vi "Validate Sequence File.vi"(10 "Path":path) -> (1 "Test Sequence":T1[](array[typedef]), 3 "Valid?":bool)   [LabVIEW 2015]
uses:
  Test Sequence Action.ctl
  Valve Action Enum.ctl
  Sequence File IO/Test Sequence Trigger.ctl
  Sequence File IO/Single Test Sequence.ctl
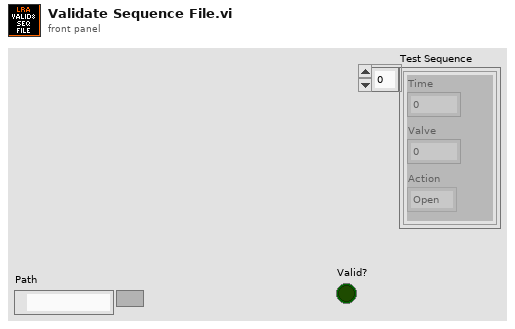
[diagram p1: front panel]
types:
  T1 = typedef "Test Sequence Action.ctl" = cluster{"Time":u32, "Valve":u32, "Action":T2}
  T2 = typedef "Valve Action Enum.ctl" = enum16{"Open", "Close"}
  T3 = typedef "Single Test Sequence.ctl" = cluster{"Actions":T1[], "Triggers":T4[]}
  T4 = typedef "Test Sequence Trigger.ctl" = cluster{"Begin Time (ms)":dbl, "End Time(ms)":dbl, "Sensor":enum16{""}, "Min Value":dbl, "Max Value":dbl}
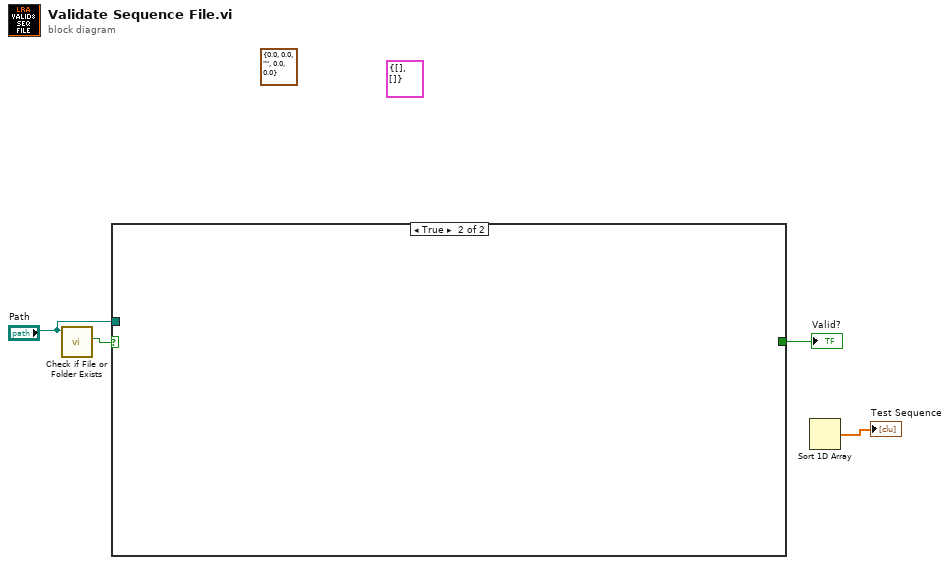
[diagram p0: block diagram]
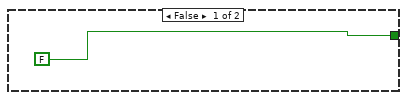
[diagram p2: hidden frame]
diagram:
  (unwired) T3 {"Actions"=[], "Triggers"=[]} ("Cluster")
  (unwired) T4 {"Begin Time (ms)"=0.0, "End Time(ms)"=0.0, "Sensor"=enum."", "Min Value"=0.0, "Max Value"=0.0}
  n1 = call <vilib>:"Check if File or Folder Exists.vi"("path"="Path") -> ("file or folder exists?"=w4:bool)  [unwired: 8 in, 2 out]
  n2 = case shown="True" w4 {
    tunnel: [FALSE _] -> w3
    tunnel: "Path" -> [_ _]
    frame False {
    }
    frame True {
    }
  }
  "Valid?" <- w3
  n3 = Sort 1D Array() -> (sorted array=→"Test Sequence":dbl[])  [unwired: 1 in]
